vi "GetDeviceVariableChoices.vi"(8 "error in (no error)":errorcluster, 10 "element":string, 11 "Device/Devicetype name\n/Plotter.id/ScanName#":string) -> (0 "error IO":errorcluster, 3 "Choiches[]":string[](array[string]))   [LabVIEW 2020]
uses:
  Shared/MySQL/Preset Query Enum.ctl
panel:
  out "data":string[][](table)
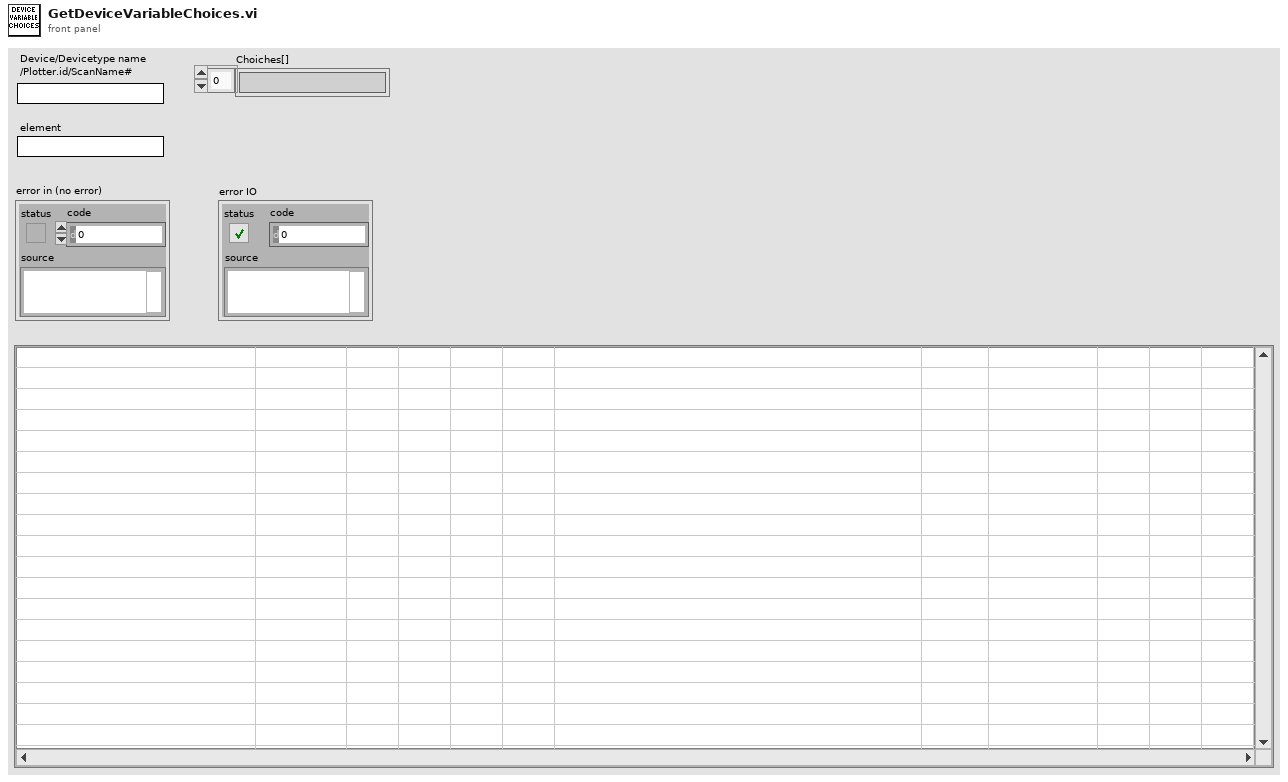
[diagram p1: front panel]
types:
  T1 = typedef "Preset Query Enum.ctl" = enum16{"Get Locations", "Get all IPs and MACs", "Get classes", "Get expt variables to set at scanstart for particular device", "Get expt devices and variables with start values", "Get expt devices and variables (with data to get)", "Get expt devices with data to get", "Get Expt devices and GUIs", "Get all devices basic properties", "Get Virtual Devices Core Info", "Get Expt names", "Get experiment basic properties", "Get experiment alarm variables", "Get MC Ports", "Get device network comm port", "Get devicetype lvclass path", "Get basic device properties", "Get Init Order", "Get all setable variables of a device", "Get device variable aliases", "Get force values of all settable variables", "Get all variables of a devicetype", "Get all variables of a device", "Get plotter details", "Get Saved Scans", "Get Scan Info", "GetGeneralGUIs", "Get expt for plotter", "Get plotter IDs from expt", "Get all devices", "Get all Virtual Devices", "Get all aliases", "Get variable and device info for Virtual Device", "GetItemLocatorIP", "Get IPs for GUIs", "Get DeviceType from Device", "GetLocalPortRange", "GetDevicePresetVariables", "Get Device Configuration", "GetAllPresetNames", "GetAllConfigurationNames", "GetPresetDeviceNames", "GetDeviceAliases", "GetDevicesOfClass"}
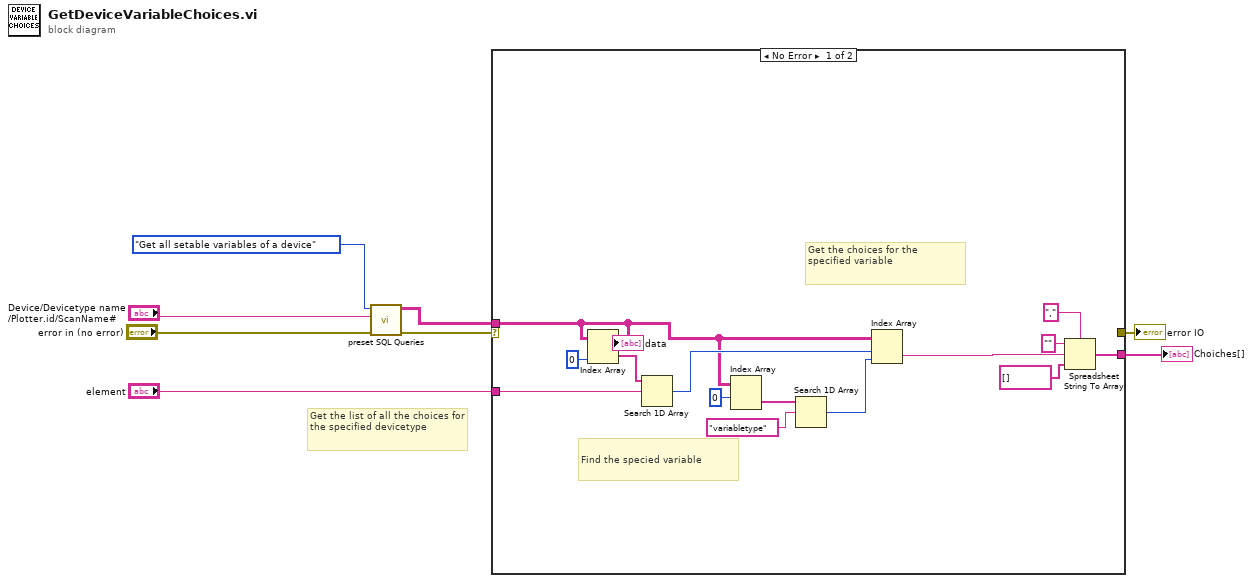
[diagram p0: block diagram]
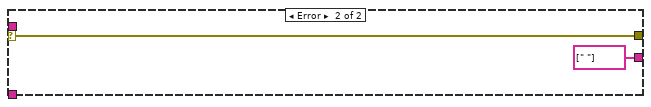
[diagram p2: hidden frame]
diagram:
  # "Get the list of all the choices for the specified devicetype"
  n1 = call "preset SQL Queries.vi"("error in (no error)"="error in (no error)", "Device/Devicetype name\n/Plotter.id/ScanName#"="Device/Devicetype name\n/Plotter.id/ScanName#", "Preset Query"=Preset_Query_Enum."Get all setable variables of a device") -> ("error out"=w5:errorcluster, "data"=w7:string[][])  [unwired: 6 in, 1 out]
  n2 = case shown="No Error" w5 {
    selector: w5 -> [_ w23]
    tunnel: [w22 string[] [" "]] -> w8
    tunnel: w7 -> [w12 _]
    tunnel: "element" -> [w16 _]
    tunnel: [_ w23] -> w4
    frame No Error {
      # "Get the choices for the specified variable"
      # "Find the specied variable"
      n3 = Index Array(array=w12, index (col)=0 ("disabled index (col)")) -> (element=w15:string[])  [unwired: 1 in]
      n4 = Search 1D Array(1D array=w15, element=w16) -> (index of element=w17:i32)  [unwired: 1 in]
      n5 = Index Array(array=w12, index (row)=0) -> (element=w10:string[])  [unwired: 1 in]
      n6 = Search 1D Array(1D array=w10, element="variabletype") -> (index of element=w13:i32)  [unwired: 1 in]
      n7 = Index Array(array=w12, index (row)=w17, index (col)=w13) -> (element=w18:string)
      n8 = Spreadsheet String To Array(delimiter (Tab)=",", format string="", spreadsheet string=w18, array type (2D Dbl)=string[] []) -> (array=w22:string[])
      "data" <- w12
    }
    frame Error {
    }
  }
  "Choiches[]" <- w8
  "error IO" <- w4
